vi "Initialisieren.vi"(8 "error in (no error)":errorcluster caption="Fehler (Eingang, kein Fehler)", 11 "Steuerung PNS Eingang":refnum<class "Steuerung PNS.lvclass">) -> (0 "error out":errorcluster caption="Fehler (Ausgang)", 3 "Steuerung PNS Ausgang":refnum<class "Steuerung PNS.lvclass">)   [LabVIEW 2020, in "Steuerung PNS.lvclass"]
doc: "Schreibt die jeweiligen SteuerungsAdressen je nach Type in das Objekt (und initialisiert Regler, UsrVal und Alarme auf 0).\nRIW"
uses:
  Steuerung PNS.lvclass
  Alarme.ctl
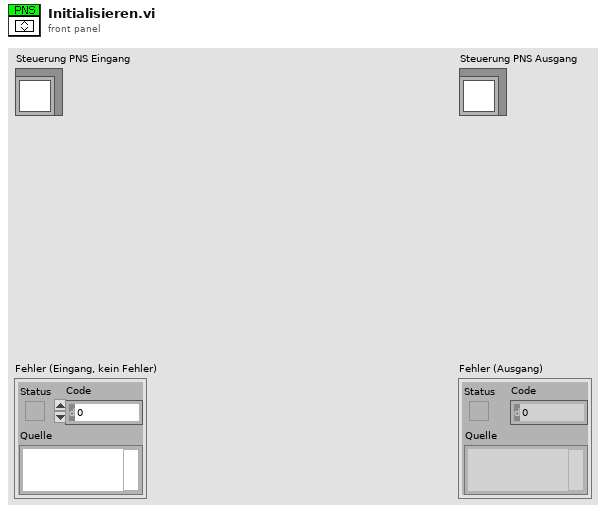
[diagram p1: front panel]
types:
  T1 = typedef "Steuerung PNS.lvclass/Alarme.ctl" = cluster{"Alarm Filter max":u16, "Alarm Filter min":u16, "Alarm Ventilplatte max":u16, "Alarm Ventilplatte min":u16, "Alarm HL1 max":u16, "Alarm HL1 min":u16, "Alarm HL2 max":u16, "Alarm HL2 min":u16, "Alarm HL3 max":u16, "Alarm HL3 min":u16, "Alarm HL4 max":u16, "Alarm HL4 min":u16, "Alarm HL5 max":u16, "Alarm HL5 min":u16, "Alarm HL6 max":u16, "Alarm HL6 min":u16}
  T2 = cluster{"Eingangs Array[0]":u16, "Eingangs Array[1]":u16, "Eingangs Array[2]":u16, "Eingangs Array[3]":u16, "Eingangs Array[4]":u16, "Eingangs Array[5]":u16}
  T3 = cluster{"Eingangs Array[0]":u16, "Eingangs Array[1]":u16, "Eingangs Array[2]":u16, "Eingangs Array[3]":u16, "Eingangs Array[4]":u16, "Eingangs Array[5]":u16}[]
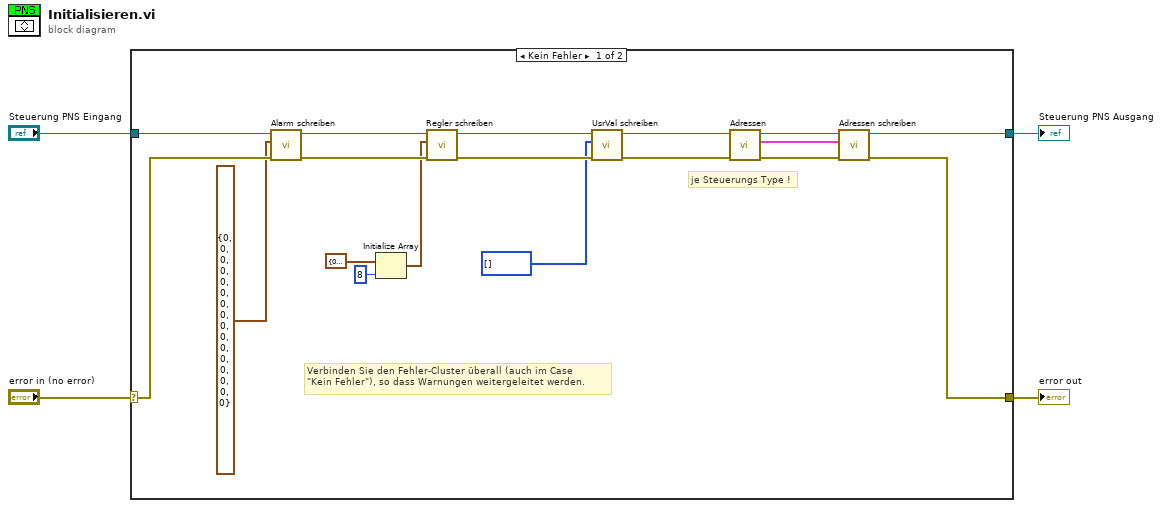
[diagram p0: block diagram]
diagram:
  n1 = case shown="Kein Fehler" "error in (no error)" {
    selector: "error in (no error)" -> [w17 w24]
    tunnel: [w7 w24] -> w3
    tunnel: [w6 w23] -> w1
    tunnel: "Steuerung PNS Eingang" -> [w22 w23]
    frame No Error {
      # "je Steuerungs Type !"
      # "Verbinden Sie den Fehler-Cluster überall (auch im Case\n\"Kein Fehler\"), so dass Warnungen weitergeleitet werden."
      n2 = call-dynamic "Alarm schreiben.vi"("error in (no error)"=w17, "Alarm"=T1 {"Alarm Filter max"=0, "Alarm Filter min"=0, "Alarm Ventilplatte max"=0, "Alarm Ventilplatte min"=0, "Alarm HL1 max"=0, "Alarm HL1 min"=0, "Alarm HL2 max"=0, "Alarm HL2 min"=0, "Alarm HL3 max"=0, "Alarm HL3 min"=0, "Alarm HL4 max"=0, "Alarm HL4 min"=0, "Alarm HL5 max"=0, "Alarm HL5 min"=0, "Alarm HL6 max"=0, "Alarm HL6 min"=0}, "Steuerung PNS (Eingang)"=w22) -> ("error out"=w19:errorcluster, "Steuerung PNS (Ausgang)"=w21:refnum<class "Steuerung PNS.lvclass">)  [unwired: 7 in]
      n3 = Initialize Array(T2 {"Eingangs Array[0]"=0, "Eingangs Array[1]"=0, "Eingangs Array[2]"=0, "Eingangs Array[3]"=0, "Eingangs Array[4]"=0, "Eingangs Array[5]"=0} ("Eingangs Array"), 8 ("Dimension")) -> (w13:T3)
      n4 = call-dynamic "Regler schreiben.vi"("error in (no error)"=w19, "Regler"=w13, "Steuerung PNS (Eingang)"=w21) -> ("error out"=w18:errorcluster, "Steuerung PNS (Ausgang)"=w20:refnum<class "Steuerung PNS.lvclass">)  [unwired: 7 in]
      n5 = call-dynamic "UsrVal schreiben.vi"("error in (no error)"=w18, "UsrVal"=u16[] [] ("Eingangs Array"), "Steuerung PNS (Eingang)"=w20) -> ("error out"=w11:errorcluster, "Steuerung PNS (Ausgang)"=w12:refnum<class "Steuerung PNS.lvclass">)  [unwired: 7 in]
      n6 = call-dynamic "Adressen.vi"("error in (no error)"=w11, "Steuerung PNS (Eingang)"=w12) -> ("error out"=w8:errorcluster, "Adressen"=w9:cluster{i32[][], i32}, "Steuerung PNS (Ausgang)"=w10:refnum<class "Steuerung PNS.lvclass">)  [unwired: 7 in]
      n7 = call-dynamic "Adressen schreiben.vi"("error in (no error)"=w8, "Adressen"=w9, "Steuerung PNS (Eingang)"=w10) -> ("error out"=w7:errorcluster, "Steuerung PNS (Ausgang)"=w6:refnum<class "Steuerung PNS.lvclass">)  [unwired: 7 in]
    }
    frame Error {
    }
  }
  "error out" <- w3
  "Steuerung PNS Ausgang" <- w1
